vi "Change Engine Library Placeholders in project.vi"(8 "error in (no error)":errorcluster, 10 "CD Wizard - Internal Data":T1, 11 "Project file content IN":string[](array[string])) -> (0 "error out":errorcluster, 3 "Project file content OUT":string[](array[string]))   [LabVIEW 2015]
uses:
  TypDef/CD Wizard - Internal data.ctl
  TypDef/CD Wizard - Execution Mode.ctl
  TypDef/CD Wizard - Extra Page Name and GUID.ctl
  Constants/Constants TypDef/CD Engine lvlib.ctl
  Constants/CD Engine lvlib.vi
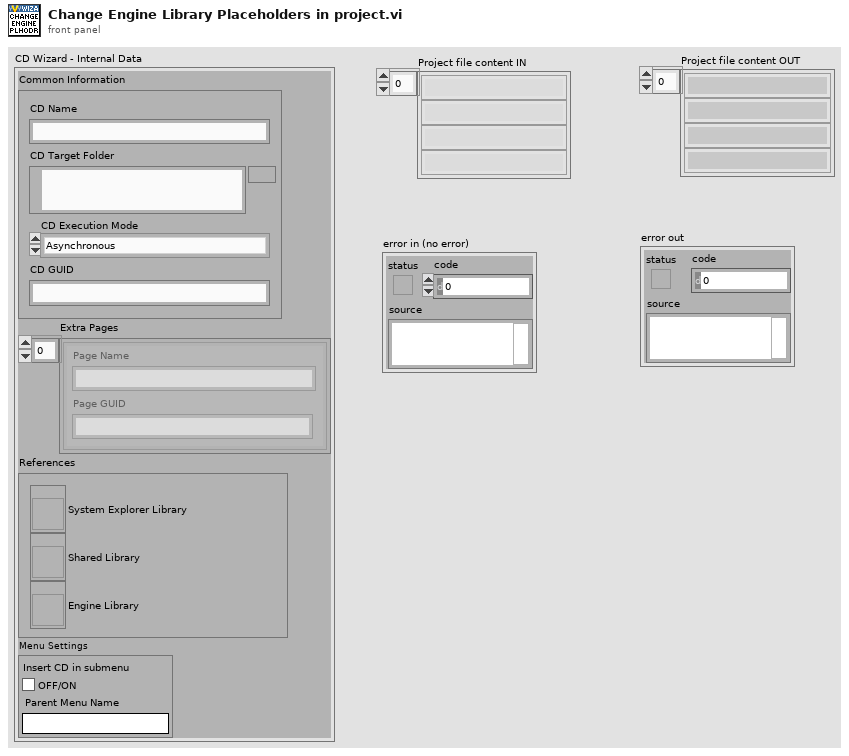
[diagram p1: front panel]
types:
  T1 = typedef "CD Wizard - Internal data.ctl" = cluster{"Common Information":cluster{"CD Name":string, "CD Target Folder":path, "CD Execution Mode":T2, "CD GUID":string}, "Extra Pages":T3[], "References":cluster{"System Explorer Library":refnum<vi>, "Shared Library":refnum<vi>, "Engine Library":refnum<vi>}, "Menu Settings":cluster{"Insert CD in submenu":bool, "Parent Menu Name":string}}
  T2 = typedef "CD Wizard - Execution Mode.ctl" = enum16{"Asynchronous", "Inline HW Interface", "Inline Model Interface", "Inline Timing and Sync", "Asynchronous Timing and Sync"}
  T3 = typedef "CD Wizard - Extra Page Name and GUID.ctl" = cluster{"Page Name":string, "Page GUID":string}
  T4 = typedef "CD Engine lvlib.ctl" = enum16{"LibraryFileName", "LibraryFolderName", "Engine.FolderName", "Engine.Init.FolderName", "Engine.Run.FolderName", "Engine.Shutdown.FolderName", "Types.FolderName", "Engine.RT Driver VI.TemplatePath", "Engine.RT Driver VI.FileName"}
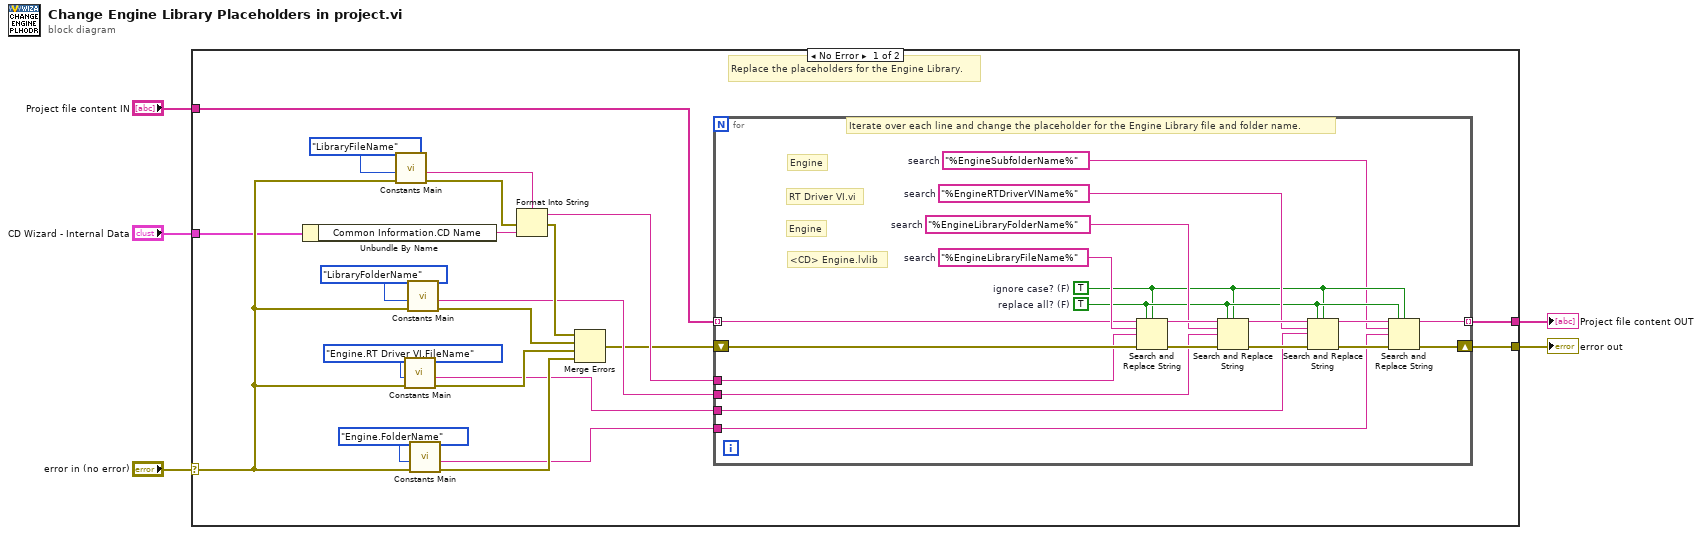
[diagram p0: block diagram]
diagram:
  n1 = case shown="No Error" "error in (no error)" {
    selector: "error in (no error)" -> [w8 w48]
    tunnel: [w26 w48] -> w5
    tunnel: [w25 w47] -> w4
    tunnel: "CD Wizard - Internal Data" -> [w7 _]
    tunnel: "Project file content IN" -> [w6 w47]
    frame No Error {
      # "Replace the placeholders for the Engine Library."
      n2 = Unbundle By Name(w7) -> ("Common Information.CD Name"=w22:string)
      n3 = call-poly "Constants Main.vi"("error in (no error)"=w8, "Action"=CD_Engine_lvlib."LibraryFileName") -> ("error out"=w23:errorcluster, "Output"=w24:string)  [unwired: 8 in]
      n4 = call-poly "Constants Main.vi"("error in (no error)"=w8, "Action"=CD_Engine_lvlib."Engine.RT Driver VI.FileName") -> ("error out"=w15:errorcluster, "Output"=w11:string)  [unwired: 8 in]
      n5 = call-poly "Constants Main.vi"("error in (no error)"=w8, "Action"=CD_Engine_lvlib."LibraryFolderName") -> ("error out"=w16:errorcluster, "Output"=w12:string)  [unwired: 8 in]
      n6 = call-poly "Constants Main.vi"("error in (no error)"=w8, "Action"=CD_Engine_lvlib."Engine.FolderName") -> ("error out"=w14:errorcluster, "Output"=w10:string)  [unwired: 8 in]
      n7 = Format Into String(format string=w24, error in=w23, w22) -> (resulting string=w13:string, error out=w17:errorcluster)  [unwired: 1 in]
      n8 = Merge Errors(w17, w16, w15, w14) -> (w9:errorcluster)
      n9 = for {
        tunnel: w6 -> [w45] mode=indexing
        shift-right: [w36] -> w26
        shift-left: w9 -> [w31]
        tunnel: [w37] -> w25 mode=indexing
        tunnel: w13 -> [w30]
        tunnel: w12 -> [w29]
        tunnel: w11 -> [w28]
        tunnel: w10 -> [w27]
        w35 = "%EngineSubfolderName%"  # search
        w41 = "%EngineRTDriverVIName%"  # search
        w43 = "%EngineLibraryFolderName%"  # search
        w38 = TRUE  # ignore case? (F)
        w39 = TRUE  # replace all? (F)
        w46 = "%EngineLibraryFileName%"  # search
        # "Engine"
        # "RT Driver VI.vi"
        # "Engine"
        # "<CD> Engine.lvlib"
        # "Iterate over each line and change the placeholder for the Engine Library file and folder name."
        n10 = Search and Replace String(replace all?=w39, case sensitive?=w38, input string=w45, search string=w46, replace string=w30, error in=w31) -> (result string=w44:string, error out=w33:errorcluster)  [unwired: 2 in, 2 out]
        n11 = Search and Replace String(replace all?=w39, case sensitive?=w38, input string=w44, search string=w43, replace string=w29, error in=w33) -> (result string=w42:string, error out=w32:errorcluster)  [unwired: 2 in, 2 out]
        n12 = Search and Replace String(replace all?=w39, case sensitive?=w38, input string=w42, search string=w41, replace string=w28, error in=w32) -> (result string=w40:string, error out=w34:errorcluster)  [unwired: 2 in, 2 out]
        n13 = Search and Replace String(replace all?=w39, case sensitive?=w38, input string=w40, search string=w35, replace string=w27, error in=w34) -> (result string=w37:string, error out=w36:errorcluster)  [unwired: 2 in, 2 out]
      }
    }
    frame Error {
      # "Output default values."
    }
  }
  "error out" <- w5
  "Project file content OUT" <- w4
